vi "Read Build spec id.vi"(11 "ProjectItem in":refnum<class "ProjectItem.lvclass">) -> (2 "Build spec id":string, 3 "ProjectItem out":refnum<class "ProjectItem.lvclass">)   [LabVIEW 2019, in "SolutionBuilder.lvlib" / "ProjectItem.lvclass"]
uses:
  ProjectItem.lvclass
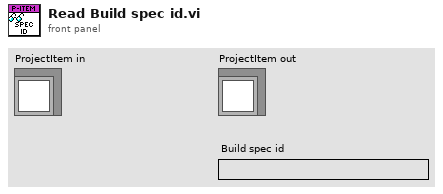
[diagram p1: front panel]
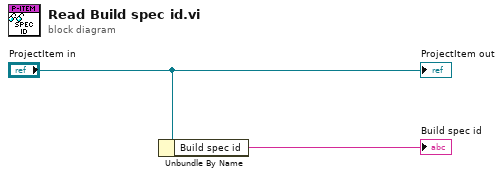
[diagram p0: block diagram]
diagram:
  n1 = Unbundle By Name("ProjectItem in") -> ("Build spec id"=→"Build spec id":string)
  "ProjectItem out" <- "ProjectItem in"
